vi "Commit Transaction.vi"(0 "connection ID in":refnum<k5>, 11 "Error In":errorcluster) -> (4 "connection ID out":refnum<k5>, 15 "Error Out":errorcluster)   [LabVIEW 2014, in "hse-db.lvlib" / "MySQL (TCP).lvlib"]
uses:
  MySQL (TCP).lvlib
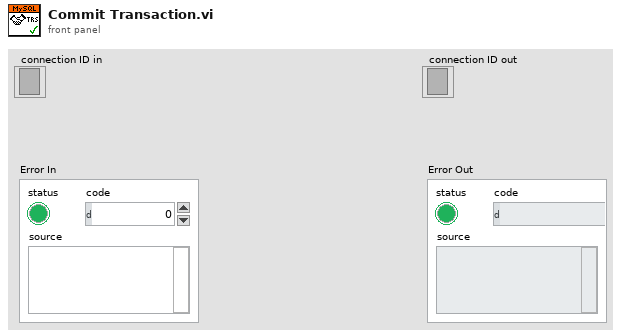
[diagram p1: front panel]
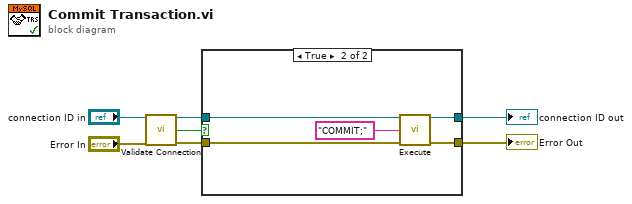
[diagram p0: block diagram]
diagram:
  n1 = call "Validate Connection.vi"("connection ID in"="connection ID in", "Error In"="Error In") -> ("connection ID out"=w4:refnum<k5>, "Valid?"=w5:bool, "Error Out"=w3:errorcluster)  [unwired: 11 in]
  n2 = case shown="True" w5 {
    tunnel: w4 -> [w9 w14]
    tunnel: w3 -> [w8 w12]
    tunnel: [w9 w13] -> w2
    tunnel: [w8 w11] -> w1
    frame False {
    }
    frame True {
      n3 = call "Execute.vi"("connection ID in"=w14, "Query"="COMMIT;", "error in (no error)"=w12) -> ("connection ID out"=w13:refnum<k5>, "error out"=w11:errorcluster)  [unwired: 7 in, 4 out]
    }
  }
  "connection ID out" <- w2
  "Error Out" <- w1
